vi "Write Meta-Data.vi"(8 "error in (no error)":errorcluster, 10 "Meta-Data":string[](array[string]), 11 "Semver in":refnum<class "Semver.lvclass">) -> (0 "error out":errorcluster, 3 "Semver out":refnum<class "Semver.lvclass">)   [LabVIEW 2017, in "Semver.lvlib" / "Semver.lvclass"]
uses:
  Semver.lvclass
  Semver.lvclass/Semver.ctl
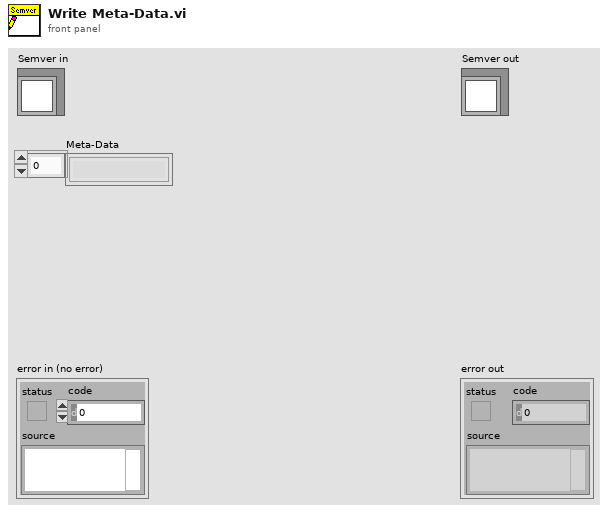
[diagram p1: front panel]
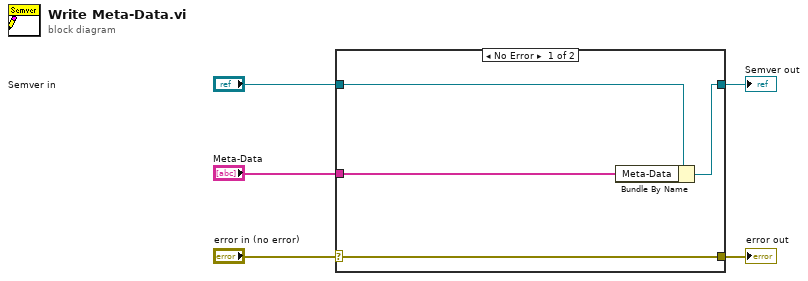
[diagram p0: block diagram]
diagram:
  n1 = case shown="No Error" "error in (no error)" {
    selector: "error in (no error)" -> [w9 w10]
    tunnel: [w9 w10] -> w4
    tunnel: [w7 w11] -> w2
    tunnel: "Semver in" -> [w8 w11]
    tunnel: "Meta-Data" -> [w6 _]
    frame No Error {
      n2 = Bundle By Name(cluster=w8, "Meta-Data"=w6) -> (w7:refnum<class "Semver.lvclass">)
    }
    frame Error {
    }
  }
  "error out" <- w4
  "Semver out" <- w2
